vi "komendahz.vi"(2 "Liniowy/logarytmiczny":bool, 3 "Amplituda":dbl, 4 "ilosc probek":u16, 5 "F min":dbl, 6 "F max":dbl) -> (0 "komendy":string[](array[string]), 1 "Czestotliwosci":dbl[](array[numeric]))   [LabVIEW 2021]
doc: "wybór komendy Hz lub kHz dla sinusa i doknanie wyboru legarytmiczny/liniowy"
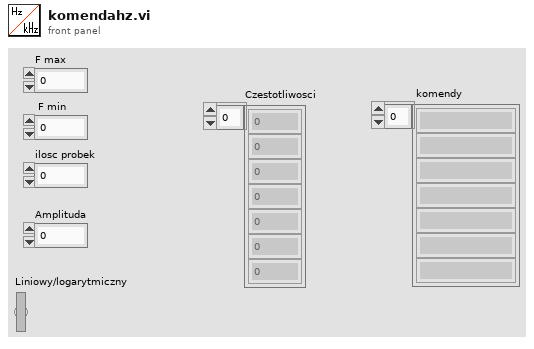
[diagram p1: front panel]
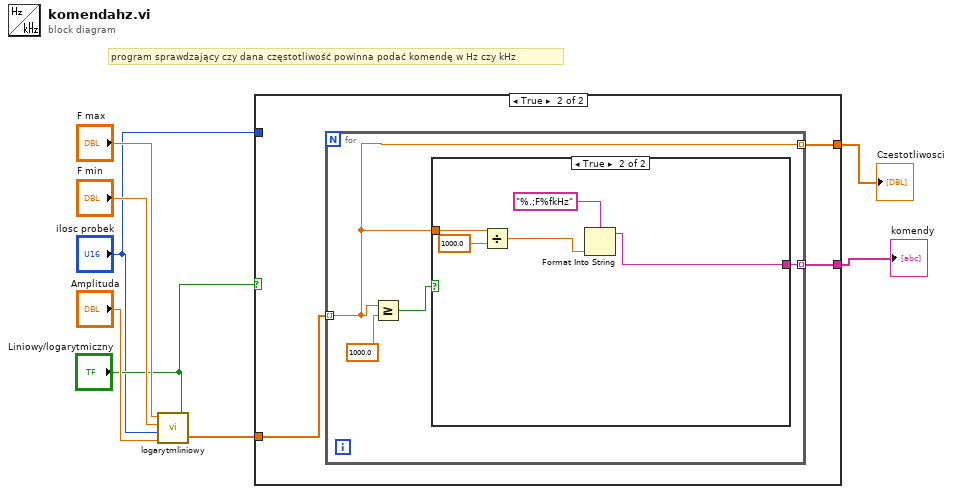
[diagram p0: block diagram]
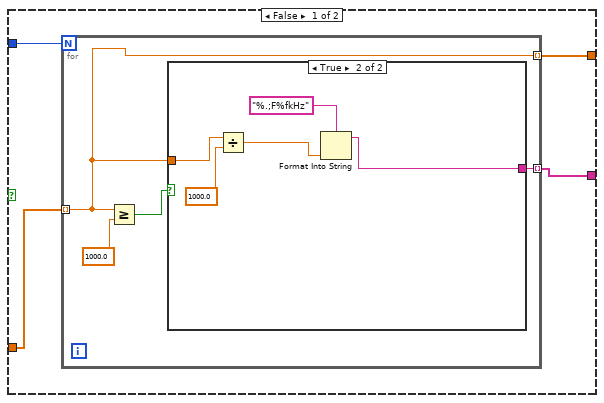
[diagram p2: hidden frame]
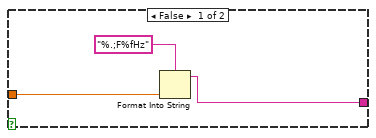
[diagram p3: hidden frame]
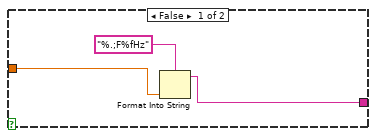
[diagram p4: hidden frame]
diagram:
  # "program sprawdzający czy dana częstotliwość powinna podać komendę w Hz czy kHz"
  n1 = call "logarytmliniowy.vi"("Liniowy/logarytmiczny"="Liniowy/logarytmiczny", "Amplituda"="Amplituda", "Ilosc probek"="ilosc probek", "F min"="F min", "F max"="F max") -> ("Czestotliwosc"=w4:dbl[])
  n2 = case shown="True" "Liniowy/logarytmiczny" {
    tunnel: w4 -> [w12 w27]
    tunnel: [w10 w26] -> w1
    tunnel: [w11 w25] -> w3
    tunnel: "ilosc probek" -> [w9 _]
    frame False {
      n3 = for {
        N: w9 -> [_]
        tunnel: [w14] -> w10 mode=indexing
        tunnel: w12 -> [w13] mode=indexing
        tunnel: [w13] -> w11 mode=indexing
        n4 = Greater Or Equal?(x=w13, y=1000.0) -> (x >= y?=w15:bool)
        n5 = case shown="True" w15 {
          tunnel: [w18 w21] -> w14
          tunnel: w13 -> [w17 w20]
          frame False {
            n6 = Format Into String(format string="%.;F%fHz", w17) -> (resulting string=w18:string)  [unwired: 2 in, 1 out]
          }
          frame True {
            n7 = Divide(x=w20, y=1000.0) -> (x/y=w23:dbl)
            n8 = Format Into String(format string="%.;F%fkHz", w23) -> (resulting string=w21:string)  [unwired: 2 in, 1 out]
          }
        }
      }
    }
    frame True {
      n9 = for {
        tunnel: w27 -> [w28] mode=indexing
        tunnel: [w29] -> w26 mode=indexing
        tunnel: [w28] -> w25 mode=indexing
        n10 = Greater Or Equal?(x=w28, y=1000.0) -> (x >= y?=w30:bool)
        n11 = case shown="True" w30 {
          tunnel: w28 -> [w34 w39]
          tunnel: [w32 w35] -> w29
          frame False {
            n12 = Format Into String(format string="%.;F%fHz", w34) -> (resulting string=w32:string)  [unwired: 2 in, 1 out]
          }
          frame True {
            n13 = Divide(x=w39, y=1000.0) -> (x/y=w37:dbl)
            n14 = Format Into String(format string="%.;F%fkHz", w37) -> (resulting string=w35:string)  [unwired: 2 in, 1 out]
          }
        }
      }
    }
  }
  "Czestotliwosci" <- w3
  "komendy" <- w1
